vi "delta_ae_guidance (SubVI).vi"(6 "Boolean":bool, 8 "Guidance gains":dbl[][](array[numeric]), 9 "k_acc":cluster{"lat_acc_mod":dbl, "up_acc":dbl}, 10 "Time":T1, 11 "e(i+1)":dbl[](array[numeric])) -> (3 "Delta azi_ele":dbl[](array[numeric]))   [LabVIEW 2017]
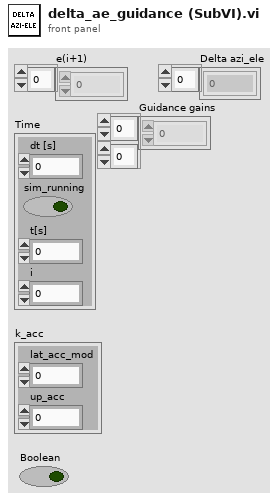
[diagram p1: front panel]
types:
  T1 = cluster{"dt [s]":dbl, "sim_running":bool, "t[s]":dbl, "i":i32}
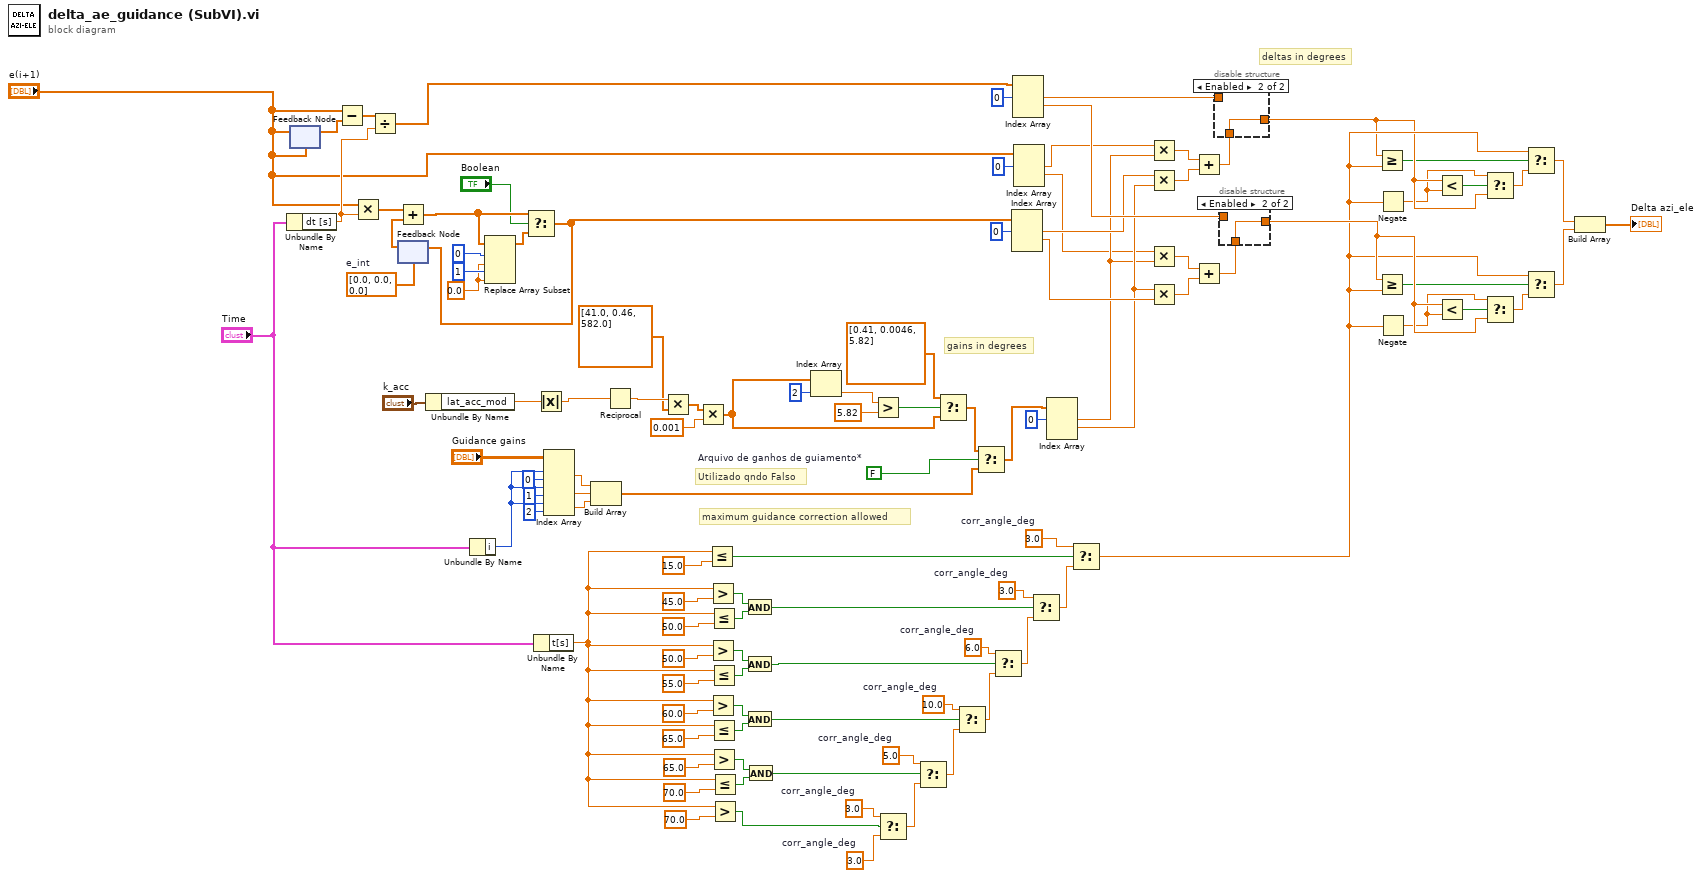
[diagram p0: block diagram]
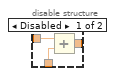
[diagram p2: hidden frame]
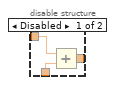
[diagram p3: hidden frame]
diagram:
  w2 = FALSE  # Arquivo de ganhos de guiamento*
  w107 = 0.0 ("new element/subarray")
  w86 = 3.0  # corr_angle_deg
  w87 = 3.0  # corr_angle_deg
  w82 = 5.0  # corr_angle_deg
  w60 = 10.0  # corr_angle_deg
  w58 = 6.0  # corr_angle_deg
  w56 = 3.0  # corr_angle_deg
  w55 = 3.0  # corr_angle_deg
  w105 = dbl[] [0.0, 0.0, 0.0]  # e_int
  # "Utilizado qndo Falso"
  # "maximum guidance correction allowed"
  # "deltas in degrees"
  # "gains in degrees"
  n1 = Unbundle By Name("Time") -> ("dt [s]"=w23:dbl)
  n2 = feedback #1("e(i+1)") -> (w21:dbl[])
  n3 = feedback-in #1("e(i+1)") -> ()
  n4 = Subtract(x="e(i+1)", y=w21) -> (x-y=w22:dbl[])
  n5 = Multiply(x="e(i+1)", y=w23) -> (x*y=w20:dbl[])
  n6 = Divide(x=w22, y=w23) -> (x/y=w39:dbl[])
  n7 = feedback #2(w105) -> (w19:dbl[])
  n8 = Add(x=w20, y=w19) -> (x+y=w109:dbl[])
  n9 = Unbundle By Name("k_acc") -> ("lat_acc_mod"=w18:dbl)
  n10 = Unbundle By Name("Time") -> ("i"=w14:i32)
  n11 = Replace Array Subset(array=w109, new element #1=w107, index #1=0 ("index"), new element #2=w107, index #2=1 ("index")) -> (w110:dbl[])
  n12 = Select(t=w109, s="Boolean", f=w110) -> (s? t:f=w16:dbl[])
  n13 = feedback-in #2(w16) -> ()
  n14 = Unbundle By Name("Time") -> ("t[s]"=w85:dbl)
  n15 = Absolute Value(x=w18) -> (abs(x)=w17:dbl)
  n16 = Index Array(array="Guidance gains", index (row) #1=w14, index (col) #1=0 ("disabled index (col)"), index (row) #2=w14, index (col) #2=1 ("disabled index (col)"), index (row) #3=w14, index (col) #3=2 ("disabled index (col)")) -> (element #1=w8:dbl, element #2=w7:dbl, element #3=w6:dbl)
  n17 = Build Array(w8, w7, w6) -> (w3:dbl[])
  n18 = Reciprocal(x=w17) -> (1/x=w25:dbl)
  n19 = Multiply(x=w25, y=dbl[] [41.0, 0.46, 582.0]) -> (x*y=w27:dbl[])
  n20 = Multiply(x=w27, y=0.001) -> (x*y=w32:dbl[])
  n21 = Less Or Equal?(x=w85, y=15.0) -> (x <= y?=w54:bool)
  n22 = Greater?(x=w85, y=45.0) -> (0:w64:bool)
  n23 = Greater?(x=w85, y=50.0) -> (0:w68:bool)
  n24 = Greater?(x=w85, y=60.0) -> (0:w73:bool)
  n25 = Less Or Equal?(x=w85, y=50.0) -> (x <= y?=w65:bool)
  n26 = Less Or Equal?(x=w85, y=55.0) -> (x <= y?=w67:bool)
  n27 = Less Or Equal?(x=w85, y=65.0) -> (x <= y?=w74:bool)
  n28 = Greater?(x=w85, y=65.0) -> (0:w76:bool)
  n29 = Less Or Equal?(x=w85, y=70.0) -> (x <= y?=w75:bool)
  n30 = Greater?(x=w85, y=70.0) -> (0:w89:bool)
  n31 = And(x=w64, y=w65) -> (x .and. y?=w66:bool)
  n32 = And(x=w68, y=w67) -> (x .and. y?=w80:bool)
  n33 = And(x=w73, y=w74) -> (x .and. y?=w81:bool)
  n34 = And(x=w76, y=w75) -> (x .and. y?=w83:bool)
  n35 = Index Array(array=w32, index=2) -> (element=w29:dbl)
  n36 = Greater?(x=w29, y=5.82) -> (0:w31:bool)
  n37 = Select(t=w87, s=w89, f=w86) -> (s? t:f=w88:dbl)
  n38 = Select(t=w82, s=w83, f=w88) -> (s? t:f=w84:dbl)
  n39 = Select(t=dbl[] [0.41, 0.0046, 5.82], s=w31, f=w32) -> (s? t:f=w4:dbl[])
  n40 = Select(t=w60, s=w81, f=w84) -> (s? t:f=w61:dbl)
  n41 = Select(t=w4, s=w2, f=w3) -> (s? t:f=w1:dbl[])
  n42 = Select(t=w58, s=w80, f=w61) -> (s? t:f=w59:dbl)
  n43 = Index Array(array=w16, index #1=0 ("index")) -> (element #1=w42:dbl, element #2=w48:dbl)  [unwired: 2 in, 1 out]
  n44 = Index Array(array=w39, index #1=0 ("index")) -> (element #1=w46:dbl, element #2=w51:dbl)  [unwired: 2 in, 1 out]
  n45 = Index Array(array="e(i+1)", index #1=0 ("index")) -> (element #1=w38:dbl, element #2=w40:dbl)  [unwired: 2 in, 1 out]
  n46 = Select(t=w56, s=w66, f=w59) -> (s? t:f=w57:dbl)
  n47 = Index Array(array=w1, index #1=0 ("index")) -> (element #1=w41:dbl, element #2=w47:dbl)  [unwired: 2 in, 1 out]
  n48 = Select(t=w55, s=w54, f=w57) -> (s? t:f=w99:dbl)
  n49 = Multiply(x=w38, y=w41) -> (x*y=w43:dbl)
  n50 = Multiply(x=w42, y=w47) -> (x*y=w44:dbl)
  n51 = Multiply(x=w40, y=w41) -> (x*y=w49:dbl)
  n52 = Multiply(x=w47, y=w48) -> (x*y=w50:dbl)
  n53 = Add(x=w43, y=w44) -> (x+y=w45:dbl)
  n54 = Add(x=w49, y=w50) -> (x+y=w52:dbl)
  n55 = disable-structure shown="Enabled" {
    disable-tunnel: [w113 w114] -> w94
    disable-tunnel: w46 -> [w112 _]
    disable-tunnel: w45 -> [w111 w114]
    frame Disabled {
      n56 = Add(x=w112, y=w111) -> (x+y=w113:dbl)
    }
    frame Enabled {
    }
  }
  n57 = disable-structure shown="Enabled" {
    disable-tunnel: [w117 w118] -> w100
    disable-tunnel: w52 -> [w116 w118]
    disable-tunnel: w51 -> [w115 _]
    frame Disabled {
      n58 = Add(x=w115, y=w116) -> (x+y=w117:dbl)
    }
    frame Enabled {
    }
  }
  n59 = Greater Or Equal?(x=w94, y=w99) -> (x >= y?=w90:bool)
  n60 = Greater Or Equal?(x=w100, y=w99) -> (x >= y?=w98:bool)
  n61 = Negate(x=w99) -> (-x=w93:dbl)
  n62 = Negate(x=w99) -> (-x=w95:dbl)
  n63 = Less?(x=w94, y=w93) -> (x < y?=w91:bool)
  n64 = Less?(x=w100, y=w95) -> (x < y?=w97:bool)
  n65 = Select(t=w93, s=w91, f=w94) -> (s? t:f=w92:dbl)
  n66 = Select(t=w95, s=w97, f=w100) -> (s? t:f=w96:dbl)
  n67 = Select(t=w99, s=w90, f=w92) -> (s? t:f=w101:dbl)
  n68 = Select(t=w99, s=w98, f=w96) -> (s? t:f=w102:dbl)
  n69 = Build Array(w101, w102) -> (→"Delta azi_ele":dbl[])
